vi "Elapsed Time Global.vi"(7 "Write (F)":bool, 9 "Ticks IN":dbl[](array[numeric]), 10 "Tick Divider":dbl format="%#_13g", 11 "Initial Times IN":dbl[](array[numeric])) -> (3 "Elapsed Times":string[](array[string]))   [LabVIEW 2019]
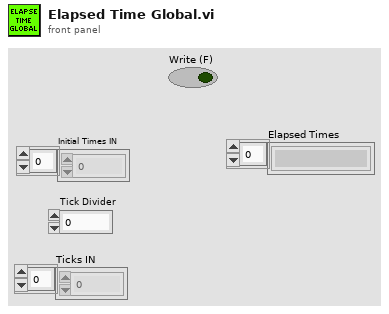
[diagram p1: front panel]
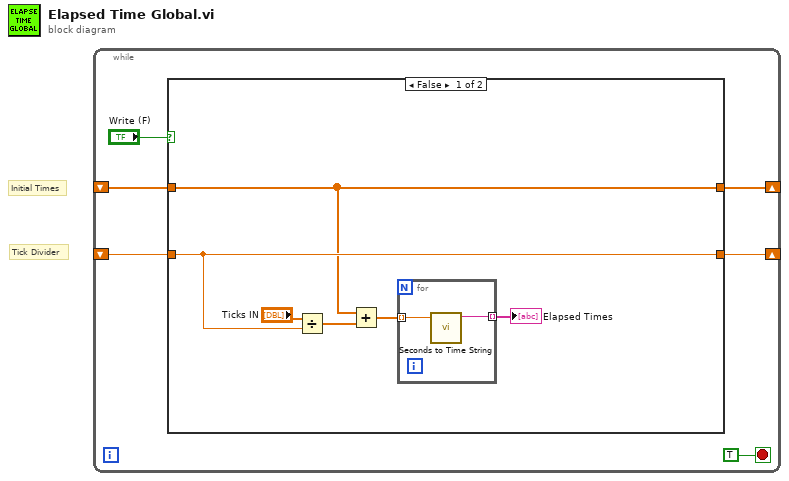
[diagram p0: block diagram]
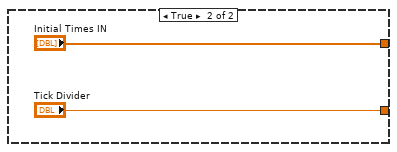
[diagram p2: hidden frame]
diagram:
  # "Tick Divider"
  # "Initial Times"
  n1 = while {
    shift-right: [w4] -> _
    shift-left: _ -> [w3]
    shift-right: [w2] -> _
    shift-left: _ -> [w1]
    stop <- TRUE stop-if-true
    n2 = case shown="False" "Write (F)" {
      tunnel: [w9 "Initial Times IN"] -> w4
      tunnel: w3 -> [w9 _]
      tunnel: [w12 "Tick Divider"] -> w2
      tunnel: w1 -> [w12 _]
      frame False {
        n3 = Divide(x="Ticks IN", y=w12) -> (x/y=w10:dbl[])
        n4 = Add(x=w9, y=w10) -> (x+y=w8:dbl[])
        n5 = for {
          tunnel: w8 -> [w14] mode=indexing
          tunnel: [w13] -> w7 mode=indexing
          n6 = call "Seconds to Time String.vi"("Seconds"=w14) -> ("Time String"=w13:string)  [unwired: 10 in]
        }
        "Elapsed Times" <- w7
      }
      frame True {
      }
    }
  }
